vi "lab_5.vi"() -> ()   [LabVIEW 2020]
uses:
  <instrlib>/Agilent 34401/Public/Data/Read (Multiple Points).vi
  <instrlib>/Agilent 2000 3000 X-Series/Public/Data/Read Measurement (Current Value).vi
  <instrlib>/Agilent 34401/Agilent 34401.lvlib
  <instrlib>/Agilent 2000 3000 X-Series/Agilent 2000 3000 X-Series.lvlib
panel:
  out "Réservoir":dbl(slide) scale=0.0..100.0
  out "Mesures de tension terminées":bool
  out "Mesures de résistance terminées":bool
  out "Progression des mesures de tension":u8(slide) scale=0.0..100.0
  in  "Nombre de mesures de tension efficace":dbl
  in  "Amplitude du générateur":dbl step=0.1
  in  "Nombre de mesures de résistance":dbl
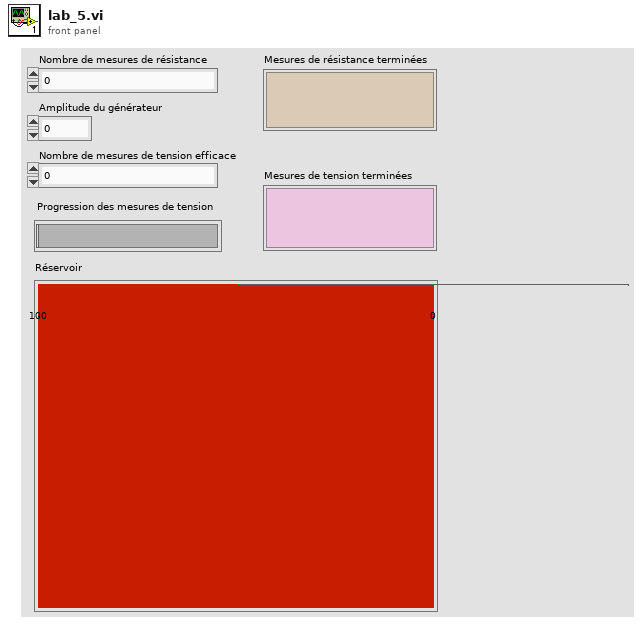
[diagram p1: front panel]
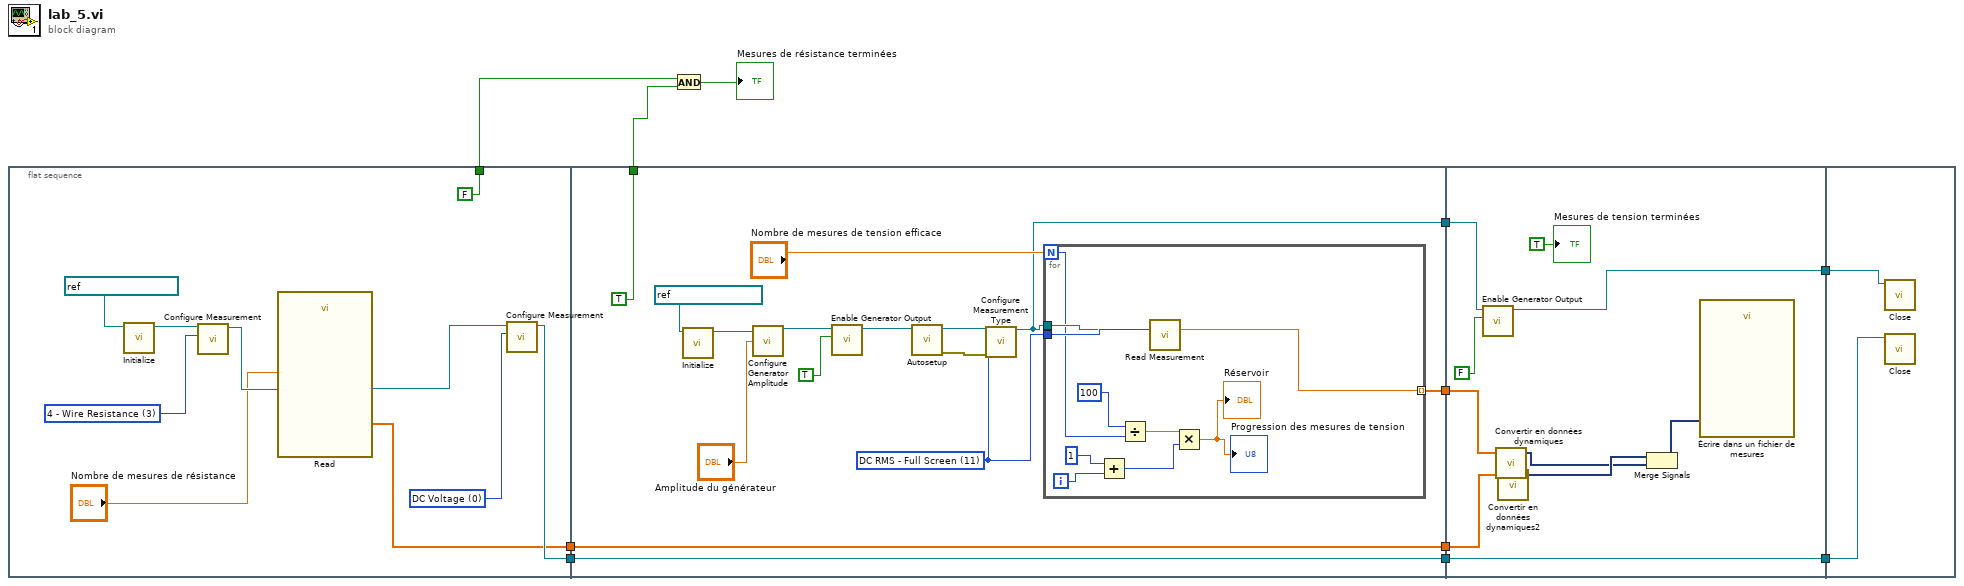
[diagram p0: block diagram]
diagram:
  n1 = flat-sequence {
    tunnel: [w13] -> w5
    tunnel: [w15] -> w4
    tunnel: [FALSE] -> w3
    tunnel: [w27] -> w11
    tunnel: [w26] -> w10
    tunnel: [w25] -> w9
    tunnel: [w24] -> w6
    tunnel: w4 -> [w24]
    tunnel: w5 -> [w25]
    tunnel: [TRUE ("Booléen")] -> w1
    tunnel: w11 -> [w55]
    tunnel: w10 -> [w54]
    tunnel: w9 -> [w52]
    tunnel: [w51] -> w8
    tunnel: [w50] -> w7
    tunnel: w6 -> [w50]
    tunnel: w8 -> [w58]
    tunnel: w7 -> [w57]
    frame #0 {
      w16 = u16 0 items=["DC Voltage", "AC Voltage", "2 - Wire Resistance", "4 - Wire Resistance", "DC Current", "AC Current", "Frequency", "Period", "Continuity", "Diode Checking", "VDC:VDC Ratio", "Temperature", "Capacitance"] ("Function (0: DC Voltage)")
      w20 = u16 3 items=["DC Voltage", "AC Voltage", "2 - Wire Resistance", "4 - Wire Resistance", "DC Current", "AC Current", "Frequency", "Period", "Continuity", "Diode Checking", "VDC:VDC Ratio", "Temperature", "Capacitance"] ("Function (0: DC Voltage)")
      n2 = call <instrlib>:"Initialize.vi"("VISA resource name"=refnum<visa-resource-name> "GPIB0::22::INSTR") -> ("VISA resource name out"=w21:refnum<visa-resource-name>)  [unwired: 9 in, 1 out]
      n3 = call <instrlib>:"Configure Measurement.vi"("Function (0: DC Voltage)"=w20, "VISA resource name"=w21) -> ("VISA resource name out"=w19:refnum<visa-resource-name>)  [unwired: 8 in, 1 out]
      n4 = call-poly <instrlib>:"Read.vi"("Sample Count (1)"="Nombre de mesures de résistance", "VISA resource name"=w19) -> ("Measurements"=w13:dbl[], "VISA resource name out"=w17:refnum<visa-resource-name>)  [unwired: 7 in, 1 out]
      n5 = call <instrlib>:"Configure Measurement.vi"("Function (0: DC Voltage)"=w16, "VISA resource name"=w17) -> ("VISA resource name out"=w15:refnum<visa-resource-name>)  [unwired: 8 in, 1 out]
    }
    frame #1 {
      w28 = 11 items=["Peak-Peak", "Maximum", "Mimimum", "Amplitude", "Top", "Base", "Overshoot", "Preshoot", "Average - N Cycles", "Average - Full Screen", "DC RMS - N Cycles", "DC RMS - Full Screen", "AC RMS - N Cycles", "AC RMS - Full Screen (Std Dev)", "Ratio", "Period", "Frequency", "Counter", "+Width", "-Width", "Burst Width", "Duty Cycle", "Rise Time", "Fall Time", "Delay", "Phase", "X minY", "X maxY", "Positive Pulse Count", "Negative Pulse Count", "Raising Edge Count", "Falling Edge Count", "Area - N Cycle", "Area - Full Screen"] ("Measurement Type (0: Peak-Peak)")
      n6 = call <instrlib>:"Initialize.vi"("VISA resource name"=refnum<visa-resource-name> "GPIB0::7::INSTR") -> ("VISA resource name out"=w36:refnum<visa-resource-name>)  [unwired: 9 in, 1 out]
      n7 = call <instrlib>:"Configure Generator Amplitude.vi"("VISA resource name"=w36, "Amplitude (1.0 V)"="Amplitude du générateur") -> ("VISA resource name out"=w34:refnum<visa-resource-name>)  [unwired: 12 in, 1 out]
      n8 = call <instrlib>:"Enable Generator Output.vi"("Enable Output (F: Disable)"=TRUE, "VISA resource name"=w34) -> ("VISA resource name out"=w33:refnum<visa-resource-name>)  [unwired: 8 in, 1 out]
      n9 = call <instrlib>:"Autosetup.vi"("VISA resource name"=w33) -> ("error out"=w29:errorcluster, "VISA resource name out"=w30:refnum<visa-resource-name>)  [unwired: 9 in]
      n10 = call <instrlib>:"Configure Measurement Type.vi"("VISA resource name"=w30, "Measurement Type (0: Peak-Peak)"=w28, "error in (no error)"=w29) -> ("VISA resource name out"=w27:refnum<visa-resource-name>)  [unwired: 11 in, 1 out]
      n11 = for {
        N: "Nombre de mesures de tension efficace" -> [w42]
        tunnel: w28 -> [w46]
        tunnel: w27 -> [w45]
        tunnel: [w44] -> w26 mode=indexing
        i -> [w39]
        n12 = Add(x=1, y=w39) -> (x+y=w38:i32)
        n13 = Divide(x=100, y=w42) -> (x/y=w41:dbl)
        n14 = call-poly <instrlib>:"Read Measurement.vi"("VISA resource name"=w45, "Measurement Type (0: Peak-Peak)"=w46) -> ("Result Value"=w44:dbl)  [unwired: 11 in, 2 out]
        n15 = Multiply(x=w41, y=w38) -> (x*y=→"Progression des mesures de tension" →"Réservoir":dbl)
      }
    }
    frame #2 {
      n16 = call <instrlib>:"Enable Generator Output.vi"("Enable Output (F: Disable)"=FALSE, "VISA resource name"=w55) -> ("VISA resource name out"=w51:refnum<visa-resource-name>)  [unwired: 8 in, 1 out]
      n17 = call "Convertir en données dynamiques"("Array"=w54) -> ("Dynamic Data Type"=w48:dynamicdata)  [unwired: 3 in]
      n18 = call "Convertir en données dynamiques2"("Array"=w52) -> ("Dynamic Data Type"=w49:dynamicdata)  [unwired: 3 in]
      n19 = Merge Signals(w49, w48) -> (w53:dynamicdata)
      n20 = call "Écrire dans un fichier de mesures"("Signals"=w53) -> ()  [unwired: 16 in, 3 out]
      "Mesures de tension terminées" <- TRUE ("Mesures de tension terminées")
    }
    frame #3 {
      n21 = call <instrlib>:"Close.vi"("VISA resource name"=w58) -> ()  [unwired: 10 in, 1 out]
      n22 = call <instrlib>:"Close.vi"("VISA resource name"=w57) -> ()  [unwired: 10 in, 1 out]
    }
  }
  n23 = And(x=w3, y=w1) -> (x .and. y?=→"Mesures de résistance terminées":bool)
